vi "Get Result.vi"(8 "error in (no error)":errorcluster caption="entrée d'erreur (pas d'erreur)", 11 "Actor Test (Default) en entrée":refnum<class "Actor Test (Default).lvclass">) -> (0 "error out":errorcluster caption="sortie d'erreur", 2 "Result":bool, 3 "Actor Test (Default) en sortie":refnum<class "Actor Test (Default).lvclass">)   [LabVIEW 2020, in "Library Core.lvlib" / "Actor Test (Default).lvclass"]
uses:
  Actor Test (Default).lvclass
  Actor Test (Default).lvclass/Actor Test (Default).ctl
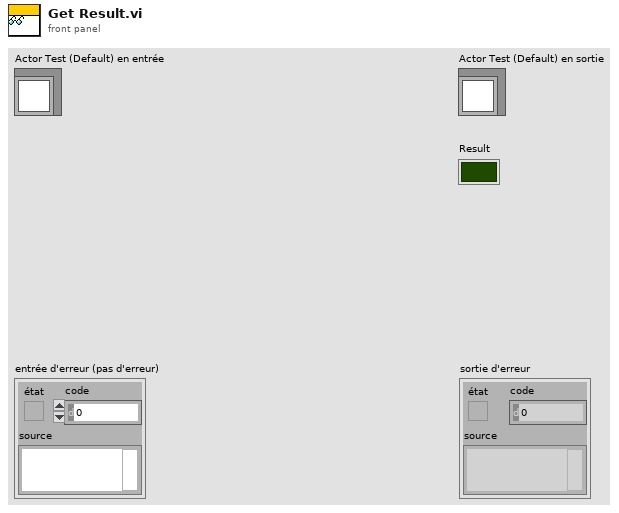
[diagram p1: front panel]
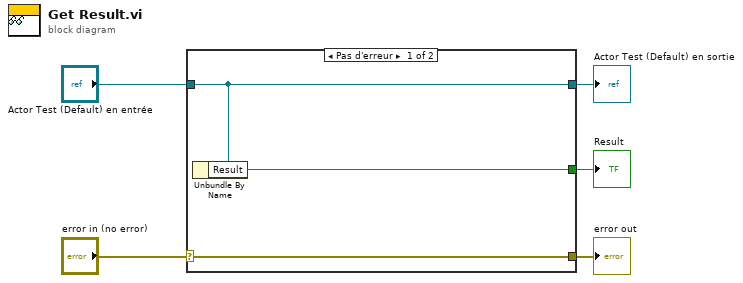
[diagram p0: block diagram]
diagram:
  n1 = case shown="Pas d'erreur" "error in (no error)" {
    selector: "error in (no error)" -> [w8 w9]
    tunnel: [w8 w9] -> w4
    tunnel: [w7 w10] -> w2
    tunnel: "Actor Test (Default) en entrée" -> [w7 w10]
    tunnel: [w6 _] -> w1
    frame No Error {
      n2 = Unbundle By Name(w7) -> ("Result"=w6:bool)
    }
    frame Error {
    }
  }
  "error out" <- w4
  "Actor Test (Default) en sortie" <- w2
  "Result" <- w1
